vi "AFG3352XGUI.contents.vi"() -> ()   [LabVIEW 2014, in "AFG3352XGUI.lvlib"]
doc: "loads all VIs into memory - required for building an application"
uses:
  AFG3352XGUI.lvlib
panel:
  out "error out":errorcluster
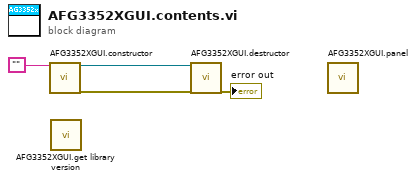
[diagram p0: block diagram]
diagram:
  n1 = call "AFG3352XGUI.constructor.vi"("name"="") -> ("i ref out"=w4:refnum<vi>, "error out"=w2:errorcluster)  [unwired: 16 in, 1 out]
  n2 = call "AFG3352XGUI.get library version.vi"() -> ()  [unwired: 1 in, 1 out]
  n3 = call "AFG3352XGUI.destructor.vi"("i ref in"=w4, "error in (no error)"=w2) -> ("error out"=→"error out":errorcluster)  [unwired: 17 in]
  n4 = call "AFG3352XGUI.panel.vi"() -> ()  [unwired: 1 in]
